vi "Chronos TDMS Read Array Size Properties.vi"(8 "error in (no error)":errorcluster, 9 "Label":string, 10 "Values":variant[](array[variant]), 11 "Properties":string[](array[string])) -> (0 "error out":errorcluster, 2 "Label dup":string, 3 "Array Dimensions":i32[](array[numeric]))   [LabVIEW 2021]
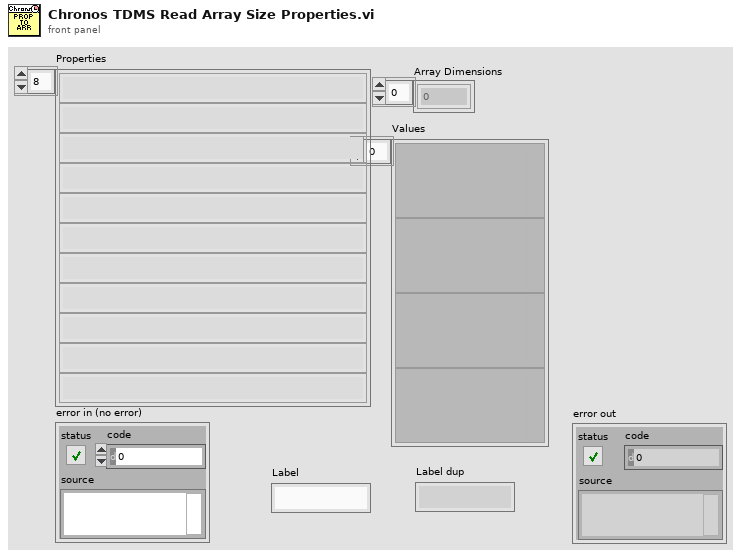
[diagram p1: front panel]
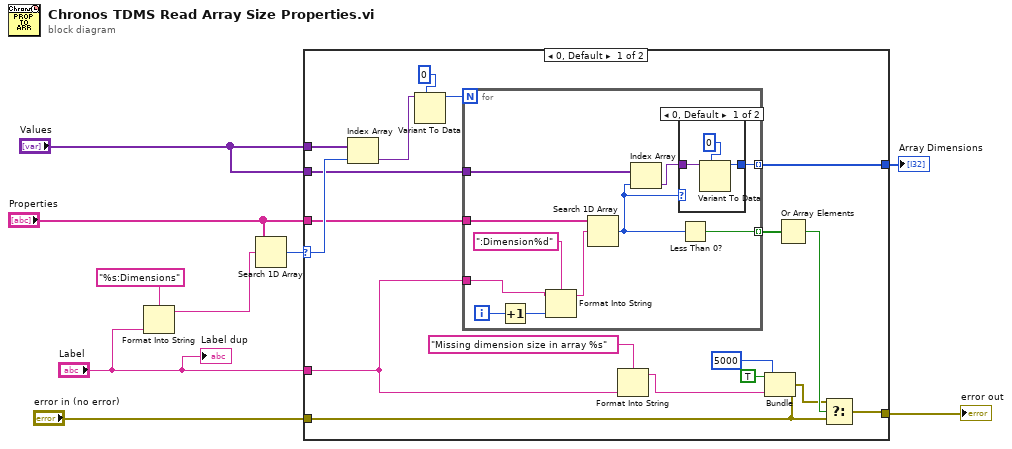
[diagram p0: block diagram]
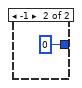
[diagram p2: hidden frame]
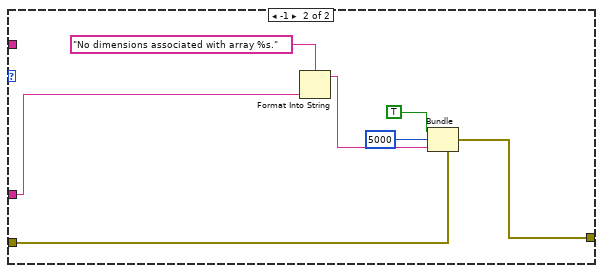
[diagram p3: hidden frame]
diagram:
  n1 = Format Into String(format string="%s:Dimensions", "Label") -> (resulting string=w8:string)  [unwired: 2 in, 1 out]
  n2 = Search 1D Array(1D array="Properties", element=w8) -> (index of element=w7:i32)  [unwired: 1 in]
  n3 = case shown="0, Default" w7 {
    selector: w7 -> [w26 _]
    tunnel: "Values" -> [w27 _]
    tunnel: "Label" -> [w15 w48]
    tunnel: "Properties" -> [w22 _]
    tunnel: "Values" -> [w21 _]
    tunnel: [w19 _] -> w4
    tunnel: "error in (no error)" -> [w14 w47]
    tunnel: [w17 w43] -> w2
    frame 0, Default {
      n4 = Index Array(array=w27, index=w26) -> (element=w24:variant)
      n5 = Variant To Data(type=0, Variant=w24) -> (data=w25:i32)  [unwired: 1 in, 1 out]
      n6 = for {
        N: w25 -> [_]
        tunnel: w15 -> [w29]
        tunnel: w22 -> [w37]
        tunnel: w21 -> [w36]
        tunnel: [w34] -> w19 mode=indexing
        tunnel: [w33] -> w20 mode=indexing
        i -> [w38]
        n7 = Increment(x=w38) -> (x+1=w31:i32)
        n8 = Format Into String(format string=":Dimension%d", initial string=w29, w31) -> (resulting string=w28:string)  [unwired: 1 in, 1 out]
        n9 = Search 1D Array(1D array=w37, element=w28) -> (index of element=w32:i32)  [unwired: 1 in]
        n10 = Index Array(array=w36, index=w32) -> (element=w35:variant)
        n11 = case shown="0, Default" w32 {
          tunnel: w35 -> [w41 _]
          tunnel: [w39 0] -> w34
          frame 0, Default {
            n12 = Variant To Data(type=0, Variant=w41) -> (data=w39:i32)  [unwired: 1 in, 1 out]
          }
          frame -1 {
          }
        }
        n13 = Less Than 0?(x=w32) -> (x < 0?=w33:bool)
      }
      n14 = Format Into String(format string="Missing dimension size in array %s", w15) -> (resulting string=w11:string)  [unwired: 2 in, 1 out]
      n15 = Bundle(cluster=w14, "status"=TRUE, "code"=5000, "source"=w11) -> (w10:errorcluster)
      n16 = Or Array Elements(Boolean array=w20) -> (logical OR=w18:bool)
      n17 = Select(t=w10, s=w18, f=w14) -> (s? t:f=w17:errorcluster)
    }
    frame -1 {
      n18 = Format Into String(format string="No dimensions associated with array %s.", w48) -> (resulting string=w45:string)  [unwired: 2 in, 1 out]
      n19 = Bundle(cluster=w47, "status"=TRUE, "code"=5000, "source"=w45) -> (w43:errorcluster)
    }
  }
  "error out" <- w2
  "Array Dimensions" <- w4
  "Label dup" <- "Label"
